vi "Install Error Codes.vi"() -> ()   [LabVIEW 2023]
panel:
  out "error out":errorcluster
  in  "Custom Error Definition File":string="MVC-Actors-errors.txt"
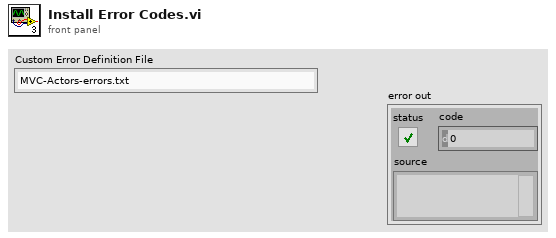
[diagram p1: front panel]
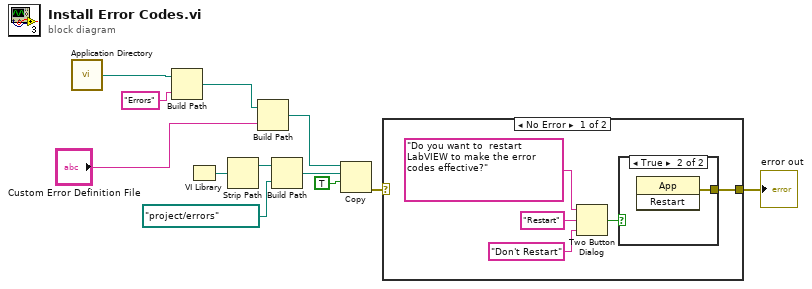
[diagram p0: block diagram]
diagram:
  n1 = call <vilib>:"Application Directory.vi"() -> ("Application Directory"=w9:path)
  n2 = Build Path(base path=w9, name or relative path="Errors" ("F button name (\"Cancel\")")) -> (appended path=w2:path)
  n3 = VI Library() -> (path=w12:path)
  n4 = Strip Path(path=w12) -> (stripped path=w10:path)  [unwired: 1 out]
  n5 = Build Path(base path=w2, name or relative path="Custom Error Definition File") -> (appended path=w7:path)
  n6 = Build Path(base path=w10, name or relative path=path "project/errors") -> (appended path=w6:path)
  n7 = Copy(9:TRUE ("overwrite (F)"), 10:w6, 11:w7) -> (0:w4:errorcluster)  [unwired: 2 in, 2 out]
  n8 = case shown="No Error" w4 {
    selector: w4 -> [_ w19]
    tunnel: [w13 w19] -> w3
    frame No Error {
      n9 = Two Button Dialog(message="Do you want to  restart LabVIEW to make the error codes effective?", 1:"Don't Restart" ("F button name (\"Cancel\")"), 2:"Restart" ("T button name (\"OK\")")) -> (T button?=w17:bool)
      n10 = case shown="True" w17 {
        tunnel: [_ w18] -> w13
        frame False {
        }
        frame True {
          n11 = invoke class="App" method="Restart"() -> (error out=w18:errorcluster)  [unwired: 3 in, 2 out]
        }
      }
    }
    frame Error {
    }
  }
  "error out" <- w3
